vi "Enter Field.vi"(7 "Field monitor":refnum<vi>, 8 "error in (no error)":errorcluster, 10 "Target field":dbl[unit], 11 "Power Supply in":refnum<class "Power Supply.lvclass">) -> (0 "error out":errorcluster, 3 "Power Supply out":refnum<class "Power Supply.lvclass">)   [LabVIEW 2009, in "Power Supply.lvclass"]
doc: "Establish an initial magnetic field - perhaps starting at zero or some other point. Use this SubVI for large (not incremental) field adjustments."
uses:
  Power Supply.lvclass
  Power Supply.lvclass/Power Supply.ctl
panel:
  in  "Dummy field monitor":dbl[unit]
  in  "Status display":refnum<vi>
  in  "resetrate?":bool
  out "canceled?":bool
  in  "cancel":bool
  out "disp":string
  out "fieldOUT":dbl[unit]
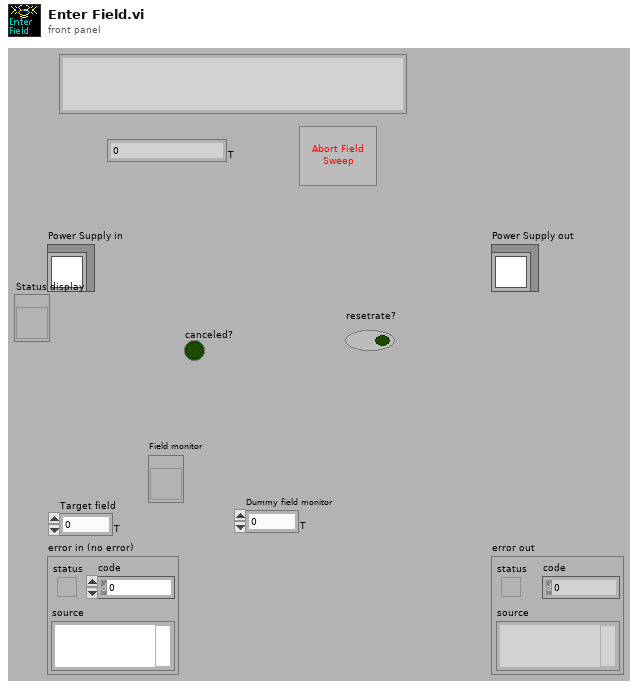
[diagram p1: front panel]
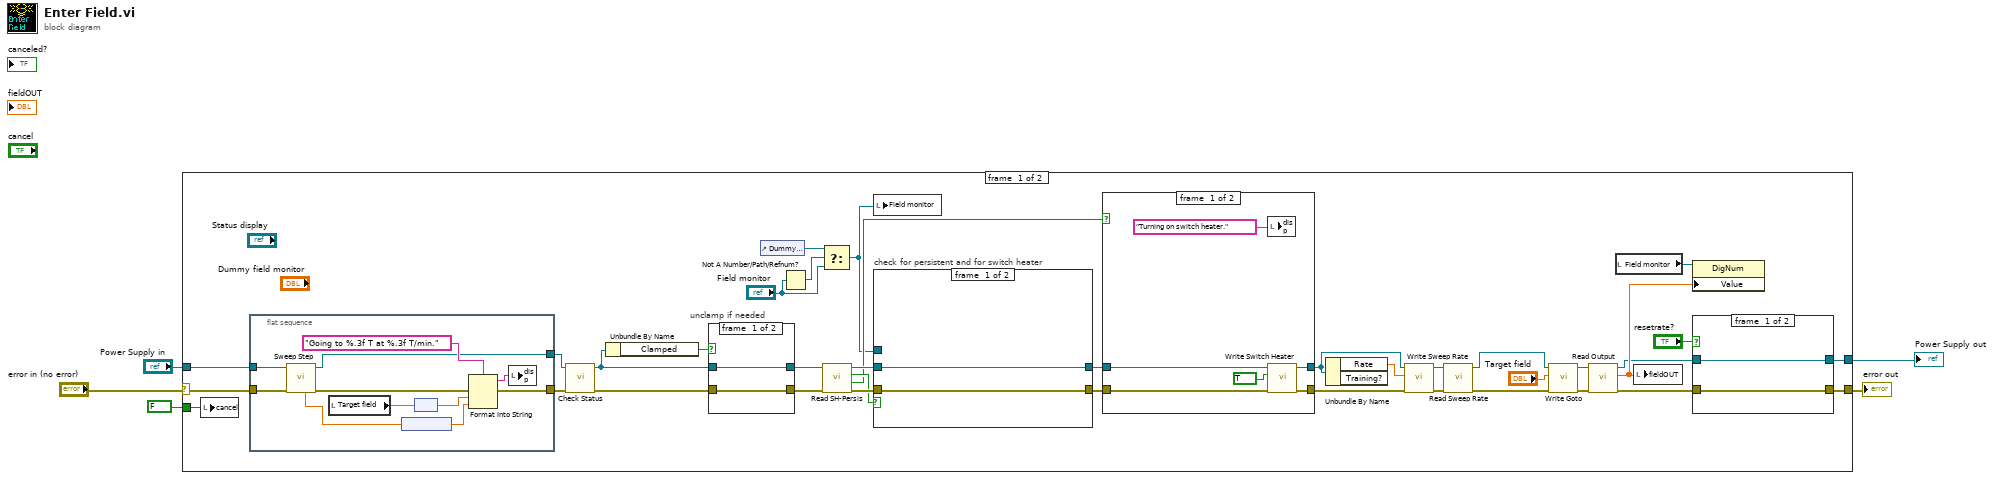
[diagram p0: block diagram]
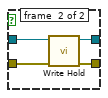
[diagram p3: hidden frame]
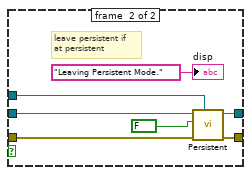
[diagram p4: hidden frame]
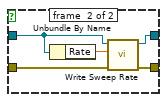
[diagram p5: hidden frame]
diagram:
  n1 = case shown="No Error" "error in (no error)" {
    selector: "error in (no error)" -> [w14 w85]
    tunnel: [w42 w85] -> w1
    tunnel: [w41 w84] -> w5
    tunnel: "Power Supply in" -> [w12 w84]
    tunnel: FALSE ("cancel") -> [w20 _]
    frame #0 {
      n2 = local write "cancel"(w20) -> ()
      n3 = flat-sequence {
        tunnel: w14 -> [w50]
        tunnel: [w51] -> w13
        tunnel: w12 -> [w43]
        tunnel: [w48] -> w11
        frame #0 {
          n4 = call-dynamic "Sweep Step.vi"("error in (no error)"=w50, "Power Supply in"=w43) -> ("error out"=w49:errorcluster, "Power Supply out"=w48:refnum<class "Power Supply.lvclass">, "rate"=w45:dbl[unit])  [unwired: 5 in, 2 out]
          n5 = local read "Target field"() -> (w47:dbl[unit])
          n6 = node(w45) -> (w44:dbl)
          n7 = node(w47) -> (w46:dbl)
          n8 = Format Into String(format string="Going to %.3f T at %.3f T/min.", error in=w49, w46, w44) -> (resulting string=w53:string, error out=w51:errorcluster)  [unwired: 1 in]
          n9 = local write "disp"(w53) -> ()
        }
      }
      n10 = call-dynamic "Check Status.vi"("error in (no error)"=w13, "Power Supply in"=w11) -> ("error out"=w27:errorcluster, "Power Supply out"=w28:refnum<class "Power Supply.lvclass">)  [unwired: 6 in, 2 out]
      n11 = Unbundle By Name(w28) -> ("Clamped"=w29:bool)
      n12 = case "unclamp if needed" shown="True" w29 {
        tunnel: w28 -> [w63 w67]
        tunnel: [w63 w66] -> w34
        tunnel: w27 -> [w62 w65]
        tunnel: [w62 w64] -> w33
        frame #0 {
        }
        frame #1 {
          n13 = call-dynamic "Write Hold.vi"("error in (no error)"=w65, "Power Supply in"=w67) -> ("error out"=w64:errorcluster, "Power Supply out"=w66:refnum<class "Power Supply.lvclass">)  [unwired: 8 in]
        }
      }
      n14 = control-ref of="Dummy field monitor"() -> (w17:refnum<vi>)
      n15 = Not A Number/Path/Refnum?(number/path/refnum="Field monitor") -> (NaN/Path/Refnum?=w19:bool)
      n16 = Select(t=w17, s=w19, f="Field monitor") -> (s? t:f=w16:refnum<vi>)
      n17 = call-dynamic "Read SH-Persis.vi"("error in (no error)"=w33, "Power Supply in"=w34) -> ("error out"=w31:errorcluster, "SHon?"=w21:bool, "pers?"=w30:bool, "Power Supply out"=w32:refnum<class "Power Supply.lvclass">)  [unwired: 4 in, 2 out]
      n18 = local write "Field monitor"(w16) -> ()
      n19 = case "check for persistent and for switch heater" shown="True" w30 {
        tunnel: w32 -> [w69 w72]
        tunnel: [w69 w73] -> w25
        tunnel: w31 -> [w68 w75]
        tunnel: [w68 w74] -> w24
        tunnel: w16 -> [_ w70]
        frame #0 {
        }
        frame #1 {
          # "leave persistent if\nat persistent"
          n20 = call-dynamic "Persistent.vi"("Field monitor ref"=w70, "error in (no error)"=w75, "Go to persistent mode?"=FALSE, "Power Supply in"=w72) -> ("error out"=w74:errorcluster, "Power Supply out"=w73:refnum<class "Power Supply.lvclass">)  [unwired: 6 in]
          "disp" <- "Leaving Persistent Mode."
        }
      }
      n21 = case shown="False" w21 {
        tunnel: w25 -> [w59 w60]
        tunnel: [w58 w60] -> w23
        tunnel: w24 -> [w57 w61]
        tunnel: [w56 w61] -> w22
        frame #0 {
          n22 = local write "disp"("Turning on switch heater." ("disp")) -> ()
          n23 = call-dynamic "Write Switch Heater.vi"("error in (no error)"=w57, "Turn SH On?"=TRUE, "Power Supply in"=w59) -> ("error out"=w56:errorcluster, "Power Supply out"=w58:refnum<class "Power Supply.lvclass">)  [unwired: 7 in]
        }
        frame #1 {
        }
      }
      n24 = Unbundle By Name(w23) -> ("Rate"=w26:dbl[unit])  [unwired: 1 out]
      n25 = call-dynamic "Write Sweep Rate.vi"("error in (no error)"=w22, "rate"=w26, "Power Supply in"=w23) -> ("error out"=w37:errorcluster, "Power Supply out"=w38:refnum<class "Power Supply.lvclass">)  [unwired: 7 in]
      n26 = call-dynamic "Read Sweep Rate.vi"("error in (no error)"=w37, "Power Supply in"=w38) -> ("error out"=w35:errorcluster, "Power Supply out"=w36:refnum<class "Power Supply.lvclass">)  [unwired: 7 in, 1 out]
      n27 = call-dynamic "Write Goto.vi"("error in (no error)"=w35, "Target"="Target field", "Power Supply in"=w36) -> ("error out"=w6:errorcluster, "Power Supply out"=w7:refnum<class "Power Supply.lvclass">)  [unwired: 7 in]
      n28 = call-dynamic "Read Output.vi"("error in (no error)"=w6, "Power Supply in"=w7) -> ("error out"=w8:errorcluster, "Field"=w10:dbl[unit], "Power Supply out"=w9:refnum<class "Power Supply.lvclass">)  [unwired: 6 in, 1 out]
      n29 = local read "Field monitor"() -> (w39:refnum<vi>)
      n30 = local write "fieldOUT"(w10) -> ()
      n31 = property class="DigNum"(reference=w39, "Value"=w10) -> ()  [unwired: 1 in, 2 out]
      n32 = case shown="True" "resetrate?" {
        tunnel: w9 -> [w78 w80]
        tunnel: w8 -> [w77 w83]
        tunnel: [w77 w82] -> w42
        tunnel: [w78 w81] -> w41
        frame #0 {
        }
        frame #1 {
          n33 = Unbundle By Name(w80) -> ("Rate"=w79:dbl[unit])
          n34 = call-dynamic "Write Sweep Rate.vi"("error in (no error)"=w83, "rate"=w79, "Power Supply in"=w80) -> ("error out"=w82:errorcluster, "Power Supply out"=w81:refnum<class "Power Supply.lvclass">)  [unwired: 7 in]
        }
      }
    }
    frame #1 {
    }
  }
  "error out" <- w1
  "Power Supply out" <- w5
